vi "ep_Get Parameters.vi"(2 "reset? (F)":bool, 5 "dt":dbl, 9 "system info in":refnum<class "EP System Info.lvclass">, 11 "error in (no error)":errorcluster) -> (4 "parameters":T1, 10 "system info out":refnum<class "EP System Info.lvclass">, 15 "error out":errorcluster)   [LabVIEW 2012, in "NI_EP_Resample_Host.lvlib"]
uses:
  <vilib>/addons/Electrical Power/PQ/Resampling/NI_EP_Resample_Host.lvlib
  <vilib>/addons/Electrical Power/PQ/Common/Classes/System Info/EP System Info.lvclass
  <vilib>/addons/Electrical Power/PQ/Resampling/Desktop/subVIs/ep_Parameters.ctl
  <vilib>/Analysis/3filter.llb/Filter Passband Type.ctl
  <vilib>/Analysis/NI_AALBase.lvlib
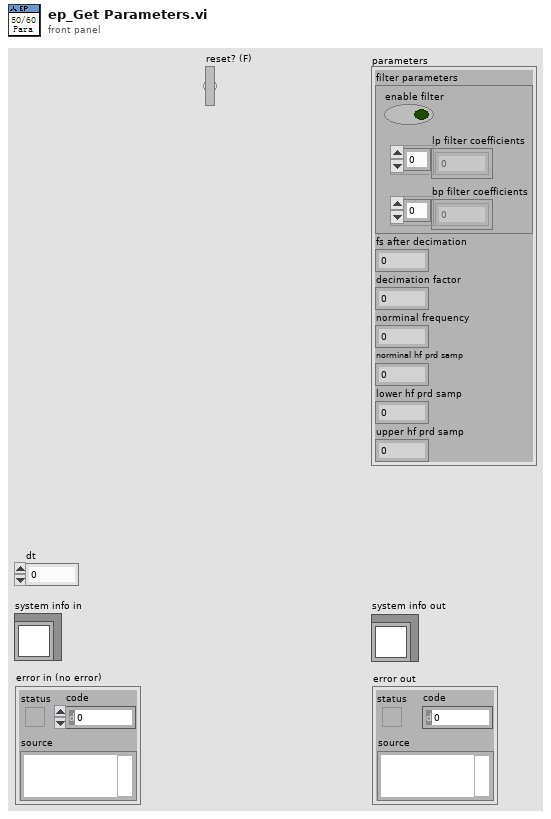
[diagram p1: front panel]
types:
  T1 = typedef "NI_EP_Resample_Host.lvlib/ep_Parameters.ctl" = cluster{"filter parameters":cluster{"enable filter":bool, "lp filter coefficients":dbl[], "bp filter coefficients":dbl[]}, "fs after decimation":dbl, "decimation factor":i32, "norminal frequency":dbl, "norminal hf prd samp":dbl, "lower hf prd samp":i32, "upper hf prd samp":i32}
  T2 = typedef "NI_AALBase.lvlib/Filter Passband Type.ctl" = enum32{"Lowpass", "Highpass", "Bandpass", "Bandstop"}
  T3 = cluster{"passband":dbl, "stopband":dbl, "dB/linear? (T: dB)":bool}
  T4 = cluster{"fpass 1":dbl, "fstop 1":dbl, "fpass 2 ":dbl, "fstop 2":dbl}
  T5 = cluster{"enable filter":bool, "filter coefficients":dbl[], "filter coefficients":dbl[]}
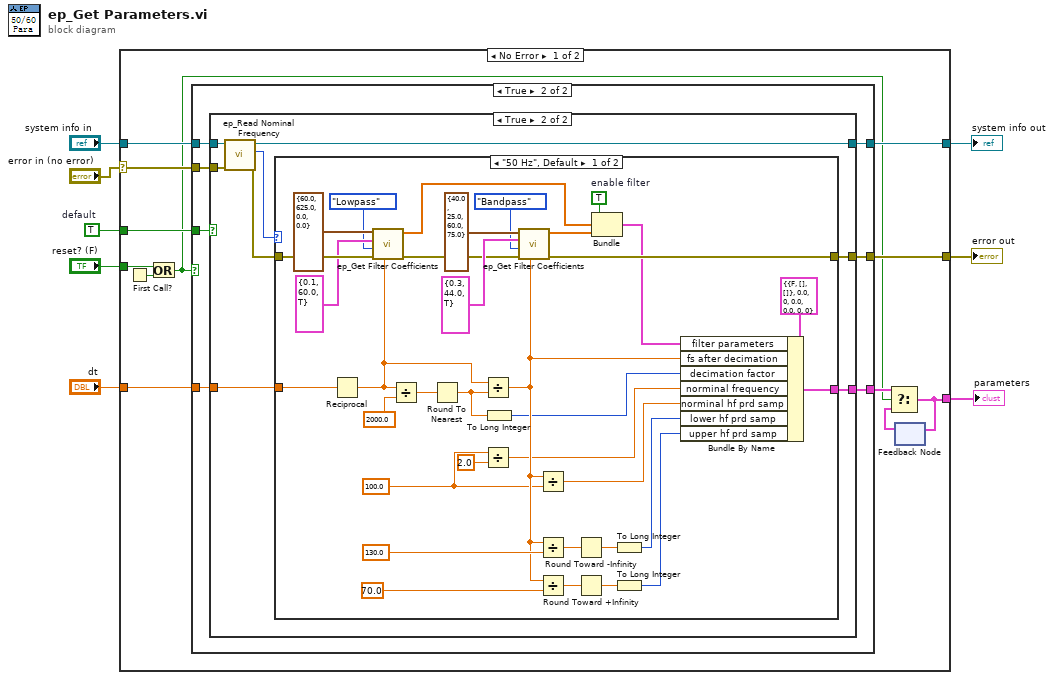
[diagram p0: block diagram]
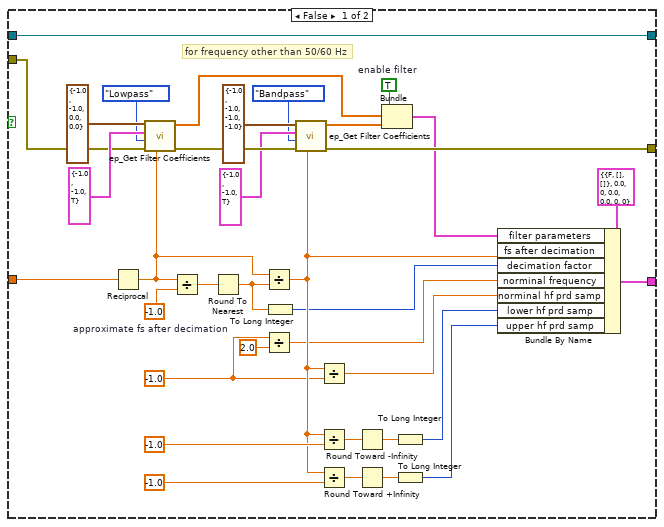
[diagram p3: hidden frame]
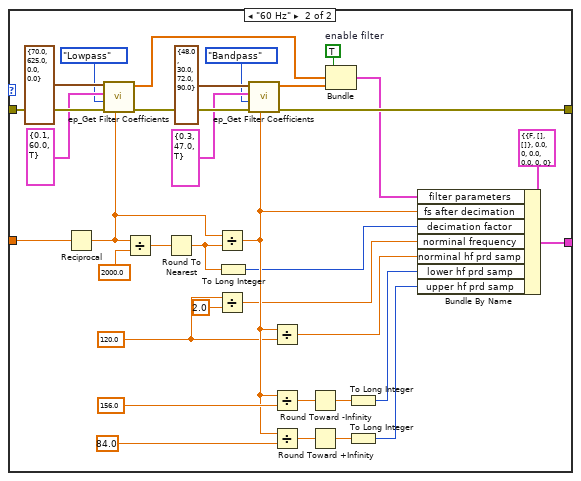
[diagram p4: hidden frame]
diagram:
  w6 = TRUE  # default
  n1 = case shown="No Error" "error in (no error)" {
    selector: "error in (no error)" -> [w15 w142]
    tunnel: "system info in" -> [w20 w141]
    tunnel: [w19 w141] -> w7
    tunnel: w6 -> [w18 _]
    tunnel: "dt" -> [w17 _]
    tunnel: [w16 w142] -> w4
    tunnel: "reset? (F)" -> [w13 _]
    tunnel: [w11 _] -> w1
    frame No Error {
      n2 = First Call?() -> (First Call?: T/F=w14:bool)
      n3 = Or(x=w13, y=w14) -> (x .or. y?=w9:bool)
      n4 = case shown="True" w9 {
        tunnel: w20 -> [w22 w29]
        tunnel: [w22 w28] -> w19
        tunnel: w18 -> [_ w27]
        tunnel: w17 -> [_ w26]
        tunnel: [w21 w25] -> w16
        tunnel: w15 -> [w21 w24]
        tunnel: [_ w23] -> w12
        frame False {
        }
        frame True {
          n5 = case shown="True" w27 {
            tunnel: w29 -> [w64 w72]
            tunnel: [w64 w71] -> w28
            tunnel: w26 -> [w39 w69]
            tunnel: w24 -> [w44 w66]
            tunnel: [w43 w68] -> w25
            tunnel: [w41 w67] -> w23
            frame False {
              w47 = TRUE  # enable filter
              w50 = -1.0  # approximate fs after decimation
              w32 = -1.0
              # "for frequency other than 50/60 Hz"
              n6 = Reciprocal(x=w39) -> (1/x=w56:dbl)
              n7 = call <vilib>:"ep_Get Filter Coefficients.vi"("fs [Hz]"=w56, "error in (no error)"=w44, "filter type"=Filter_Passband_Type."Lowpass", "ripple specs"=T3 {"passband"=-1.0, "stopband"=-1.0, "dB/linear? (T: dB)"=TRUE}, "freq specs [Hz]"=T4 {"fpass 1"=-1.0, "fstop 1"=-1.0, "fpass 2 "=0.0, "fstop 2"=0.0}) -> ("error out"=w55:errorcluster, "filter coefficients"=w46:dbl[])  [unwired: 4 in, 1 out]
              n8 = Divide(x=w56, y=w50) -> (x/y=w51:dbl)
              n9 = Round To Nearest(number=w51) -> (nearest integer value=w52:dbl)
              n10 = Divide(x=w56, y=w52) -> (x/y=w38:dbl)
              n11 = Divide(x=w32, y=2.0) -> (x/y=w36:dbl)
              n12 = To Long Integer(number=w52) -> (32bit integer=w37:i32)
              n13 = call <vilib>:"ep_Get Filter Coefficients.vi"("fs [Hz]"=w38, "error in (no error)"=w55, "filter type"=Filter_Passband_Type."Bandpass", "ripple specs"=T3 {"passband"=-1.0, "stopband"=-1.0, "dB/linear? (T: dB)"=TRUE}, "freq specs [Hz]"=T4 {"fpass 1"=-1.0, "fstop 1"=-1.0, "fpass 2 "=-1.0, "fstop 2"=-1.0}) -> ("error out"=w43:errorcluster, "filter coefficients"=w45:dbl[])  [unwired: 4 in, 1 out]
              n14 = Divide(x=w38, y=w32) -> (x/y=w35:dbl)
              n15 = Divide(x=w38, y=-1.0) -> (x/y=w61:dbl)
              n16 = Divide(x=w38, y=-1.0) -> (x/y=w63:dbl)
              n17 = Round Toward -Infinity(1:w61) -> (0:w60:dbl)
              n18 = Round Toward +Infinity(x=w63) -> (ceil(x): smallest int >= x=w62:dbl)
              n19 = Bundle("enable filter"=w47, "filter coefficients"=w46, "filter coefficients"=w45) -> (w40:T5)  [unwired: 1 in]
              n20 = To Long Integer(number=w60) -> (32bit integer=w34:i32)
              n21 = To Long Integer(number=w62) -> (32bit integer=w33:i32)
              n22 = Bundle By Name(cluster=T1 {"filter parameters"={"enable filter"=FALSE, "lp filter coefficients"=[], "bp filter coefficients"=[]}, "fs after decimation"=0.0, "decimation factor"=0, "norminal frequency"=0.0, "norminal hf prd samp"=0.0, "lower hf prd samp"=0, "upper hf prd samp"=0} ("output cluster 2"), "filter parameters"=w40, "fs after decimation"=w38, "decimation factor"=w37, "norminal frequency"=w36, "norminal hf prd samp"=w35, "lower hf prd samp"=w34, "upper hf prd samp"=w33) -> (w41:T1)
            }
            frame True {
              n23 = call <vilib>:"ep_Read Nominal Frequency.vi"("error in (no error)"=w66, "system info in"=w72) -> ("error out"=w65:errorcluster, "nominal frequency"=w70:enum16{"50 Hz", "60 Hz"}, "system info out"=w71:refnum<class "EP System Info.lvclass">)  [unwired: 6 in, 1 out]
              n24 = case shown="\"50 Hz\", Default" w70 {
                tunnel: w69 -> [w88 w107]
                tunnel: w65 -> [w95 w129]
                tunnel: [w94 w128] -> w68
                tunnel: [w90 w117] -> w67
                frame "50 Hz", Default {
                  w93 = TRUE  # enable filter
                  w76 = 100.0
                  n25 = Reciprocal(x=w88) -> (1/x=w103:dbl)
                  n26 = call <vilib>:"ep_Get Filter Coefficients.vi"("fs [Hz]"=w103, "error in (no error)"=w95, "filter type"=Filter_Passband_Type."Lowpass", "ripple specs"=T3 {"passband"=0.1, "stopband"=60.0, "dB/linear? (T: dB)"=TRUE}, "freq specs [Hz]"=T4 {"fpass 1"=60.0, "fstop 1"=625.0, "fpass 2 "=0.0, "fstop 2"=0.0}) -> ("error out"=w78:errorcluster, "filter coefficients"=w91:dbl[])  [unwired: 4 in, 1 out]
                  n27 = Divide(x=w103, y=2000.0) -> (x/y=w105:dbl)
                  n28 = Round To Nearest(number=w105) -> (nearest integer value=w104:dbl)
                  n29 = Divide(x=w103, y=w104) -> (x/y=w87:dbl)
                  n30 = Divide(x=w76, y=2.0) -> (x/y=w75:dbl)
                  n31 = To Long Integer(number=w104) -> (32bit integer=w86:i32)
                  n32 = call <vilib>:"ep_Get Filter Coefficients.vi"("fs [Hz]"=w87, "error in (no error)"=w78, "filter type"=Filter_Passband_Type."Bandpass", "ripple specs"=T3 {"passband"=0.3, "stopband"=44.0, "dB/linear? (T: dB)"=TRUE}, "freq specs [Hz]"=T4 {"fpass 1"=40.0, "fstop 1"=25.0, "fpass 2 "=60.0, "fstop 2"=75.0}) -> ("error out"=w94:errorcluster, "filter coefficients"=w92:dbl[])  [unwired: 4 in, 1 out]
                  n33 = Divide(x=w87, y=w76) -> (x/y=w85:dbl)
                  n34 = Divide(x=w87, y=130.0) -> (x/y=w98:dbl)
                  n35 = Divide(x=w87, y=70.0) -> (x/y=w96:dbl)
                  n36 = Round Toward -Infinity(1:w98) -> (0:w99:dbl)
                  n37 = Round Toward +Infinity(x=w96) -> (ceil(x): smallest int >= x=w97:dbl)
                  n38 = Bundle("enable filter"=w93, "filter coefficients"=w91, "filter coefficients"=w92) -> (w89:T5)  [unwired: 1 in]
                  n39 = To Long Integer(number=w99) -> (32bit integer=w84:i32)
                  n40 = To Long Integer(number=w97) -> (32bit integer=w83:i32)
                  n41 = Bundle By Name(cluster=T1 {"filter parameters"={"enable filter"=FALSE, "lp filter coefficients"=[], "bp filter coefficients"=[]}, "fs after decimation"=0.0, "decimation factor"=0, "norminal frequency"=0.0, "norminal hf prd samp"=0.0, "lower hf prd samp"=0, "upper hf prd samp"=0} ("output cluster 2"), "filter parameters"=w89, "fs after decimation"=w87, "decimation factor"=w86, "norminal frequency"=w75, "norminal hf prd samp"=w85, "lower hf prd samp"=w84, "upper hf prd samp"=w83) -> (w90:T1)
                }
                frame "60 Hz" {
                  w127 = TRUE  # enable filter
                  w110 = 120.0
                  n42 = Reciprocal(x=w107) -> (1/x=w133:dbl)
                  n43 = call <vilib>:"ep_Get Filter Coefficients.vi"("fs [Hz]"=w133, "error in (no error)"=w129, "filter type"=Filter_Passband_Type."Lowpass", "ripple specs"=T3 {"passband"=0.1, "stopband"=60.0, "dB/linear? (T: dB)"=TRUE}, "freq specs [Hz]"=T4 {"fpass 1"=70.0, "fstop 1"=625.0, "fpass 2 "=0.0, "fstop 2"=0.0}) -> ("error out"=w116:errorcluster, "filter coefficients"=w126:dbl[])  [unwired: 4 in, 1 out]
                  n44 = Divide(x=w133, y=2000.0) -> (x/y=w131:dbl)
                  n45 = Round To Nearest(number=w131) -> (nearest integer value=w132:dbl)
                  n46 = Divide(x=w133, y=w132) -> (x/y=w123:dbl)
                  n47 = Divide(x=w110, y=2.0) -> (x/y=w121:dbl)
                  n48 = To Long Integer(number=w132) -> (32bit integer=w122:i32)
                  n49 = call <vilib>:"ep_Get Filter Coefficients.vi"("fs [Hz]"=w123, "error in (no error)"=w116, "filter type"=Filter_Passband_Type."Bandpass", "ripple specs"=T3 {"passband"=0.3, "stopband"=47.0, "dB/linear? (T: dB)"=TRUE}, "freq specs [Hz]"=T4 {"fpass 1"=48.0, "fstop 1"=30.0, "fpass 2 "=72.0, "fstop 2"=90.0}) -> ("error out"=w128:errorcluster, "filter coefficients"=w125:dbl[])  [unwired: 4 in, 1 out]
                  n50 = Divide(x=w123, y=w110) -> (x/y=w120:dbl)
                  n51 = Divide(x=w123, y=156.0) -> (x/y=w138:dbl)
                  n52 = Divide(x=w123, y=84.0) -> (x/y=w140:dbl)
                  n53 = Round Toward -Infinity(1:w138) -> (0:w137:dbl)
                  n54 = Round Toward +Infinity(x=w140) -> (ceil(x): smallest int >= x=w139:dbl)
                  n55 = Bundle("enable filter"=w127, "filter coefficients"=w126, "filter coefficients"=w125) -> (w124:T5)  [unwired: 1 in]
                  n56 = To Long Integer(number=w137) -> (32bit integer=w119:i32)
                  n57 = To Long Integer(number=w139) -> (32bit integer=w118:i32)
                  n58 = Bundle By Name(cluster=T1 {"filter parameters"={"enable filter"=FALSE, "lp filter coefficients"=[], "bp filter coefficients"=[]}, "fs after decimation"=0.0, "decimation factor"=0, "norminal frequency"=0.0, "norminal hf prd samp"=0.0, "lower hf prd samp"=0, "upper hf prd samp"=0} ("output cluster 2"), "filter parameters"=w124, "fs after decimation"=w123, "decimation factor"=w122, "norminal frequency"=w121, "norminal hf prd samp"=w120, "lower hf prd samp"=w119, "upper hf prd samp"=w118) -> (w117:T1)
                }
              }
            }
          }
        }
      }
      n59 = feedback #1() -> (w10:T1)  [unwired: 1 in]
      n60 = Select(t=w12, s=w9, f=w10) -> (s? t:f=w11:T1)
      n61 = feedback-in #1(w11) -> ()
    }
    frame Error {
    }
  }
  "system info out" <- w7
  "error out" <- w4
  "parameters" <- w1
